vi "group Sync Read Remove Param.vi"(8 "error in (no error)":errorcluster, 10 "id":u8, 11 "group_num":i32) -> (0 "error out":errorcluster)   [LabVIEW 2022 SP3, in "dxl.lvlib"]
doc: "WINDECLSPEC void groupSyncReadRemoveParam (int group_num, uint8_t id);"
uses:
  dxl.lvlib
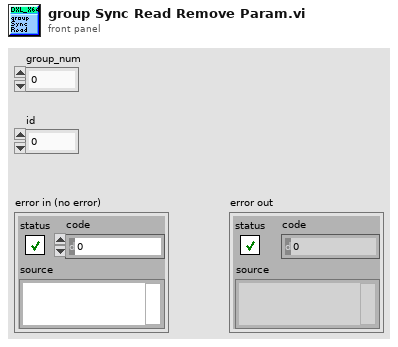
[diagram p1: front panel]
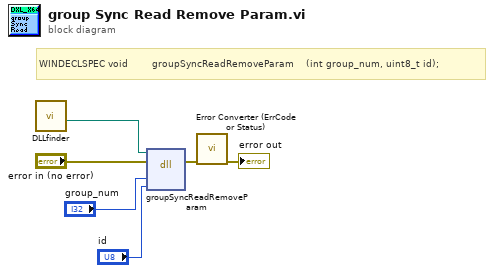
[diagram p0: block diagram]
diagram:
  # "WINDECLSPEC void        groupSyncReadRemoveParam    (int group_num, uint8_t id);"
  n1 = call "DLLfinder.vi"() -> ("File Path"=w1:path)  [unwired: 11 in]
  n2 = dll-call lib="C:/EnFlo_Software/ADAM Serial/Instrument drivers/Dynamixel/2nd attempt/Library/dxl_x64_c.*" fn="groupSyncReadRemoveParam"(path in=w1, error in="error in (no error)", "group_num"="group_num", "id"="id") -> (error out=w3:errorcluster)  [unwired: 4 in, 1 out]
  n3 = call "Error Converter (ErrCode or Status).vi"("error in (no error)"=w3) -> ("error out"=→"error out":errorcluster)  [unwired: 10 in]
